vi "Clear.vi"(8 "error in (no error)":errorcluster, 11 "Error Log in":refnum<class "Error Log.lvclass">) -> (0 "error out":errorcluster, 2 "Error Log File Path":path, 3 "Error Log out":refnum<class "Error Log.lvclass">)   [LabVIEW 2020, in "Error Log Classes.lvlib" / "Error Log.lvclass"]
uses:
  Error Log.lvclass
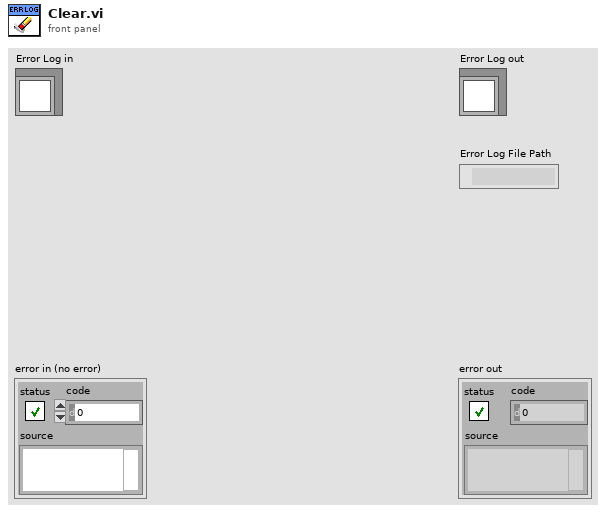
[diagram p1: front panel]
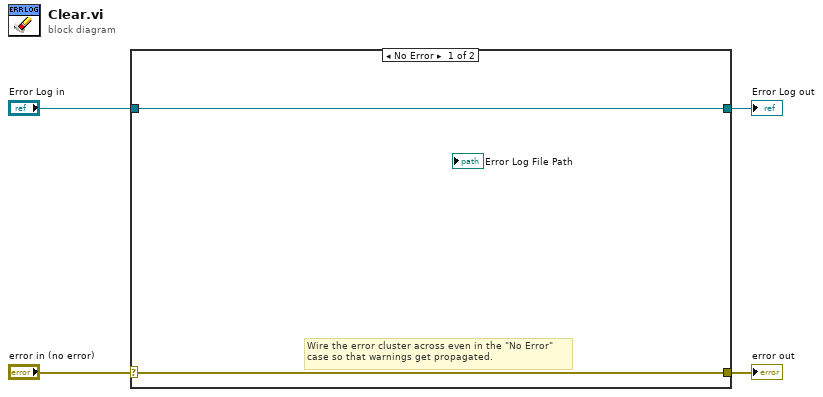
[diagram p0: block diagram]
diagram:
  n1 = case shown="No Error" "error in (no error)" {
    selector: "error in (no error)" -> [w5 w8]
    tunnel: [w5 w8] -> w3
    tunnel: [w6 w7] -> w1
    tunnel: "Error Log in" -> [w6 w7]
    frame No Error {
      # "Wire the error cluster across even in the \"No Error\"\ncase so that warnings get propagated."
    }
    frame Error {
    }
  }
  "error out" <- w3
  "Error Log out" <- w1
